vi "Stop Core.vi"(10 "final error code":i32, 11 "HardwareSetup_modle001:HardwareSetup_modle001":refnum<class "HardwareSetup_model001.lvclass">) -> (3 "HardwareSetup_modle001:HardwareSetup_modle001":refnum<class "HardwareSetup_model001.lvclass">)   [LabVIEW 2019, in "HardwareSetup_model001.lvlib" / "HardwareSetup_model001.lvclass"]
uses:
  HardwareSetup_model001.lvclass
  HardwareSetup_model001.lvclass/HardwareSetup_model001.ctl
  SystemSetup/SystemSetup/SystemSetup.lvclass
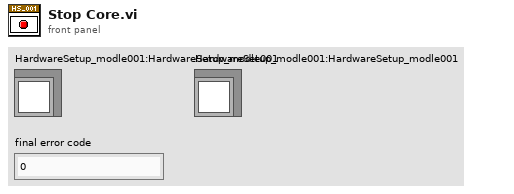
[diagram p1: front panel]
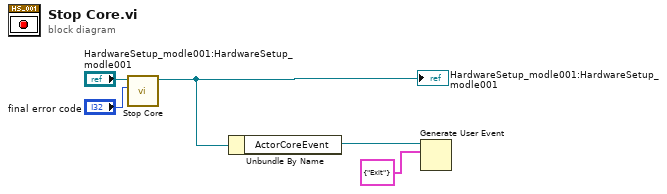
[diagram p0: block diagram]
diagram:
  n1 = call-parent "Stop Core.vi"("final error code"="final error code", "Event Source In"="HardwareSetup_modle001:HardwareSetup_modle001") -> ("Event Source Out"=w1:refnum<class "HardwareSetup_model001.lvclass">)  [unwired: 9 in]
  "HardwareSetup_modle001:HardwareSetup_modle001" <- w1
  n2 = Unbundle By Name(w1) -> ("ActorCoreEvent"=w3:refnum<user-event>)
  n3 = Generate User Event(user event=w3, event data cluster=cluster{"ActorCoreMessage":string} {"ActorCoreMessage"="Exit"} ("event data")) -> ()  [unwired: 2 in, 2 out]
